vi "stage globals.vi"() -> ()   [LabVIEW 2011]
uses:
  Stage/Move stage command.ctl
panel:
  in  "Stage name":string="Mad City Labs 1 x 1 x 1 um TTL controller"
  in  "x max (um)":ext=100.0
  out "Current Z (um)":ext=50.0 format="%_5g"
  out "Current Y (um)":ext=50.0 format="%_5g"
  out "Current X (um)":ext=50.0 format="%_5g"
  in  "Default\nstage settle time (ms)":u32=2000
  in  "Stage Calibration Factors":T1={"x cal fac UM/v"=10.0074999999999999997, "y cal fac UM/v"=10.002, "z cal fac UM/v"=9.997}
  in  "Number of field steps":i16
  in  "Field step":i16
  in  "z max (um)":ext=100.0
  in  "y max (um)":ext=100.0
  out "user event out":refnum<user-event>
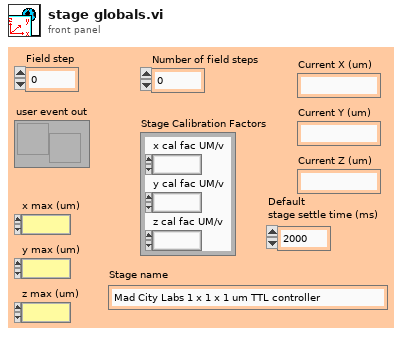
[diagram p1: front panel]
types:
  T1 = cluster{"x cal fac UM/v":ext, "y cal fac UM/v":ext, "z cal fac UM/v":ext}
diagram:
